vi "Initialize AO Channels.vi"(8 "error in (no error)":errorcluster, 11 "Instrument.Lockin":refnum<class "Instrument.Lockin.lvclass">) -> (0 "error out":errorcluster, 3 "Instrument.Lockin out":refnum<class "Instrument.Lockin.lvclass">)   [LabVIEW 2020, in "Instrument.Lockin.lvclass"]
uses:
  Instrument.Lockin.lvclass
  Instrument.Lockin.lvclass/Instrument.Lockin.ctl
  LockinDAQ/Typedefs/Function-enum.ctl
  LockinDAQ/LockinDAQ.lvclass
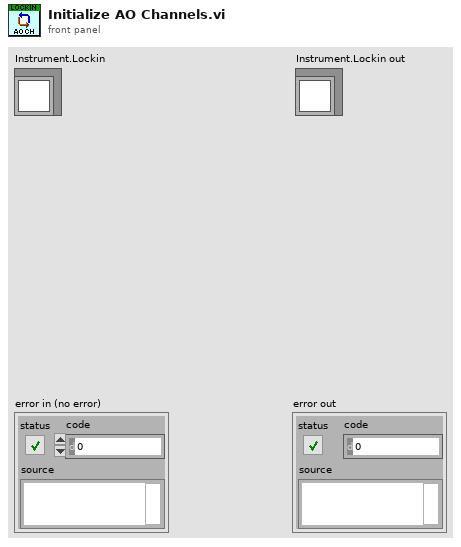
[diagram p1: front panel]
types:
  T1 = typedef "LockinDAQ.lvclass/AO-cluster.ctl" = cluster{"Ch":i32[], "Amp (V)":dbl[], "DC (V)":dbl[], "f (Hz)":dbl[], "Phase (°)":dbl[], "Function":T2[], "Sweep?":bool[]}
  T2 = typedef "LockinDAQ.lvclass/Function-enum.ctl" = enum16{"Sine", "Triangle", "Square", "Sawtooth"}
  T3 = typedef "LockinDAQ.lvclass/AO.config-array.ctl" = T4[]
  T4 = typedef "LockinDAQ.lvclass/AO.config-cluster.ctl" = cluster{"AO.channels":tag, "AO.Range":T5, "output terminal configuration":i32, "DAQ Type":T6}
  T5 = typedef "LockinDAQ.lvclass/446xAO-enum.ctl" = enum16{"±0.1 V", "±1.0 V", "±10.0 V"}
  T6 = typedef "LockinDAQ.lvclass/DAQType-enum.ctl" = enum16{"None", "USB 4431", "PXI 446x"}
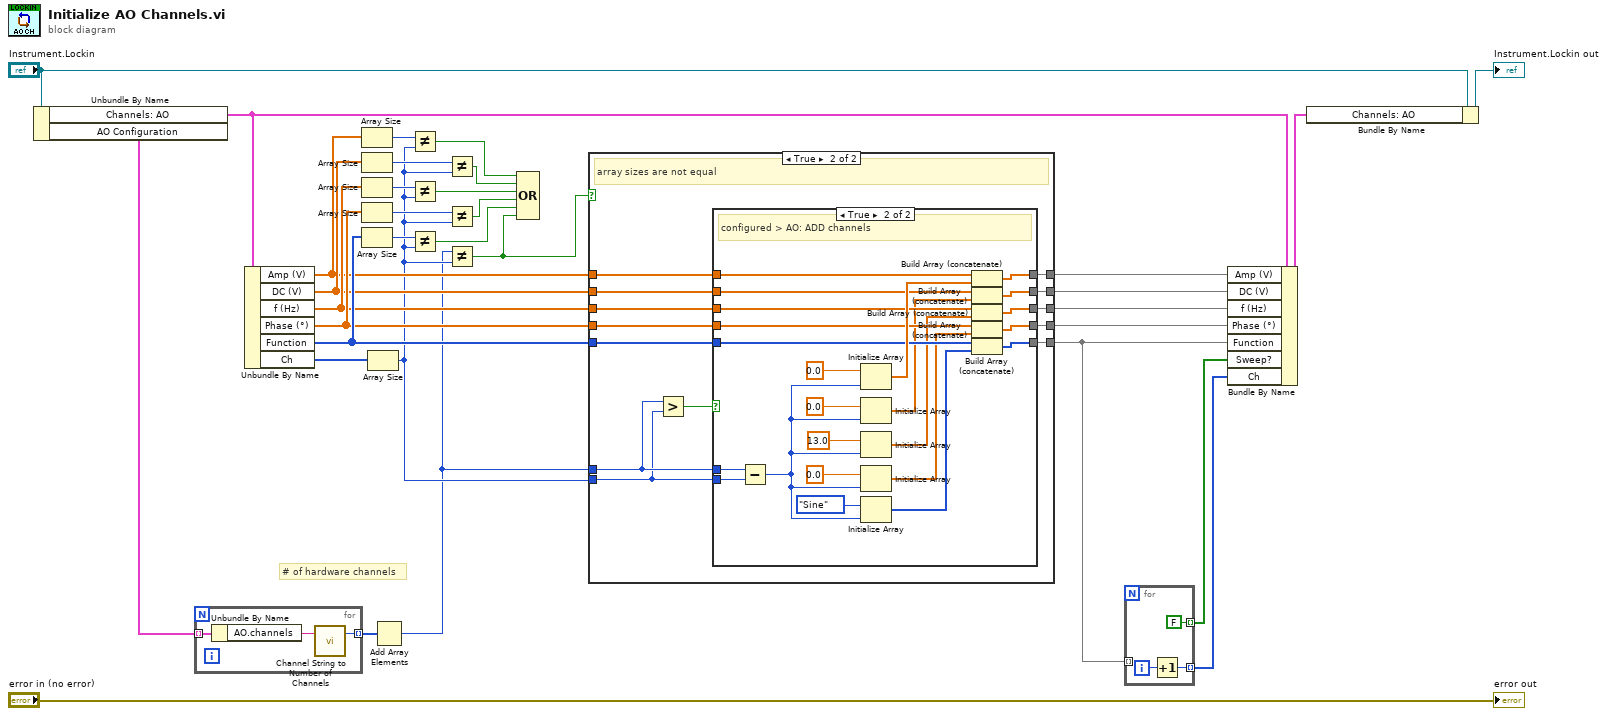
[diagram p0: block diagram]
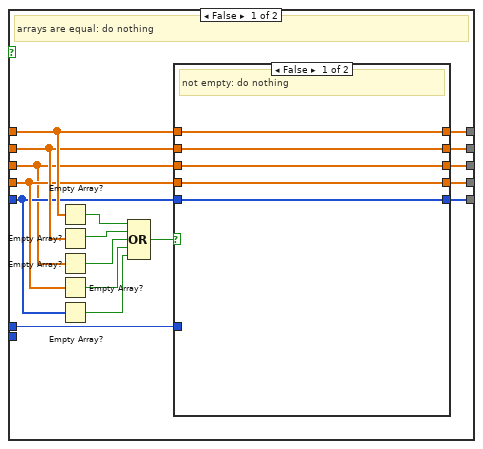
[diagram p2: hidden frame]
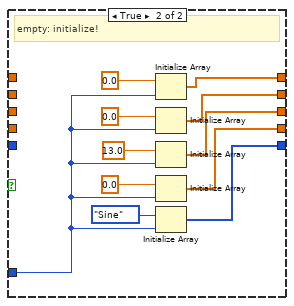
[diagram p3: hidden frame]
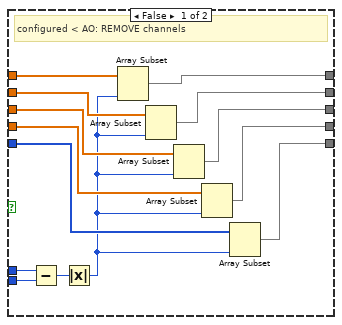
[diagram p4: hidden frame]
diagram:
  # "# of hardware channels"
  n1 = Unbundle By Name("Instrument.Lockin") -> ("Channels: AO"=w28:T1, "AO Configuration"=w5:T3)
  n2 = for {
    tunnel: w5 -> [w36] mode=indexing
    tunnel: [w35] -> w30 mode=indexing
    n3 = Unbundle By Name(w36) -> ("AO.channels"=w34:tag)
    n4 = call "Channel String to Number of Channels.vi"("Channels String"=w34) -> ("# channels"=w35:i32)  [unwired: 2 in]
  }
  n5 = Unbundle By Name(w28) -> ("Amp (V)"=w20:dbl[], "DC (V)"=w21:dbl[], "f (Hz)"=w22:dbl[], "Phase (°)"=w23:dbl[], "Function"=w24:T2[], "Ch"=w8:i32[])
  n6 = Array Size(array=w20) -> (size(s)=w19:i32)
  n7 = Array Size(array=w21) -> (size(s)=w18:i32)
  n8 = Array Size(array=w22) -> (size(s)=w17:i32)
  n9 = Array Size(array=w23) -> (size(s)=w16:i32)
  n10 = Array Size(array=w24) -> (size(s)=w15:i32)
  n11 = Array Size(array=w8) -> (size(s)=w9:i32)
  n12 = Add Array Elements(numeric array=w30) -> (sum=w4:i32)
  n13 = Not Equal?(x=w19, y=w9) -> (x != y?=w14:bool)
  n14 = Not Equal?(x=w17, y=w9) -> (x != y?=w12:bool)
  n15 = Not Equal?(x=w15, y=w9) -> (x != y?=w10:bool)
  n16 = Not Equal?(x=w18, y=w9) -> (x != y?=w13:bool)
  n17 = Not Equal?(x=w16, y=w9) -> (x != y?=w11:bool)
  n18 = Not Equal?(x=w4, y=w9) -> (x != y?=w3:bool)
  n19 = Compound Arithmetic op=OR(w14, w13, w12, w11, w10, w3) -> ()  [unwired: 1 out]
  n20 = case shown="True" w3 {
    tunnel: [w48 w75] -> w2
    tunnel: w24 -> [w42 w70]
    tunnel: [w49 w76] -> w31
    tunnel: [w47 w74] -> w32
    tunnel: w22 -> [w41 w78]
    tunnel: w21 -> [w44 w80]
    tunnel: [w45 w82] -> w33
    tunnel: w23 -> [w43 w77]
    tunnel: w20 -> [w53 w81]
    tunnel: w4 -> [w50 w72]
    tunnel: w9 -> [_ w71]
    tunnel: [w46 w79] -> w27
    frame False {
      # "arrays are equal: do nothing"
      n21 = Empty Array?(array=w53) -> (empty?=w52:bool)
      n22 = Empty Array?(array=w44) -> (empty?=w40:bool)
      n23 = Empty Array?(array=w41) -> (empty?=w39:bool)
      n24 = Empty Array?(array=w43) -> (empty?=w38:bool)
      n25 = Empty Array?(array=w42) -> (empty?=w37:bool)
      n26 = Compound Arithmetic op=OR(w52, w40, w39, w38, w37) -> (w51:bool)
      n27 = case shown="False" w51 {
        tunnel: w42 -> [w54 _]
        tunnel: w43 -> [w55 _]
        tunnel: w41 -> [w56 _]
        tunnel: w44 -> [w57 _]
        tunnel: w53 -> [w58 _]
        tunnel: w50 -> [_ w64]
        tunnel: [w55 w63] -> w49
        tunnel: [w54 w62] -> w48
        tunnel: [w56 w61] -> w47
        tunnel: [w57 w60] -> w46
        tunnel: [w58 w59] -> w45
        frame False {
          # "not empty: do nothing"
        }
        frame True {
          # "empty: initialize!"
          n28 = Initialize Array(0.0, w64) -> (w59:dbl[])
          n29 = Initialize Array(0.0, w64) -> (w60:dbl[])
          n30 = Initialize Array(13.0, w64) -> (w61:dbl[])
          n31 = Initialize Array(0.0, w64) -> (w63:dbl[])
          n32 = Initialize Array(Function-enum."Sine" ("Signal Type"), w64) -> (w62:T2[])
        }
      }
    }
    frame True {
      # "array sizes are not equal"
      n33 = Greater?(x=w72, y=w71) -> (0:w73:bool)
      n34 = case shown="True" w73 {
        tunnel: [w91 w114] -> w82
        tunnel: w81 -> [w92 w113]
        tunnel: w72 -> [w86 w111]
        tunnel: w71 -> [w85 w110]
        tunnel: w80 -> [w93 w108]
        tunnel: [w90 w107] -> w79
        tunnel: w78 -> [w94 w106]
        tunnel: w77 -> [w95 w105]
        tunnel: [w88 w104] -> w76
        tunnel: [w87 w102] -> w75
        tunnel: [w89 w97] -> w74
        tunnel: w70 -> [w96 w103]
        frame False {
          # "configured < AO: REMOVE channels"
          n35 = Subtract(x=w86, y=w85) -> (x-y=w84:i32)
          n36 = Absolute Value(x=w84) -> (abs(x)=w83:i32)
          n37 = Array Subset(array=w92, length=w83) -> (w91:dbl[])  [unwired: 1 in]
          n38 = Array Subset(array=w93, length=w83) -> (w90:dbl[])  [unwired: 1 in]
          n39 = Array Subset(array=w94, length=w83) -> (w89:dbl[])  [unwired: 1 in]
          n40 = Array Subset(array=w95, length=w83) -> (w88:dbl[])  [unwired: 1 in]
          n41 = Array Subset(array=w96, length=w83) -> (w87:T2[])  [unwired: 1 in]
        }
        frame True {
          # "configured > AO: ADD channels"
          n42 = Subtract(x=w111, y=w110) -> (x-y=w109:i32)
          n43 = Initialize Array(0.0, w109) -> (w112:dbl[])
          n44 = Initialize Array(0.0, w109) -> (w101:dbl[])
          n45 = Initialize Array(13.0, w109) -> (w100:dbl[])
          n46 = Initialize Array(0.0, w109) -> (w99:dbl[])
          n47 = Initialize Array(Function-enum."Sine" ("Signal Type"), w109) -> (w98:T2[])
          n48 = Build Array (concatenate)(w113, w112) -> (w114:dbl[])
          n49 = Build Array (concatenate)(w108, w101) -> (w107:dbl[])
          n50 = Build Array (concatenate)(w106, w100) -> (w97:dbl[])
          n51 = Build Array (concatenate)(w105, w99) -> (w104:dbl[])
          n52 = Build Array (concatenate)(w103, w98) -> (w102:T2[])
        }
      }
    }
  }
  n53 = for {
    tunnel: [w121] -> w7 mode=indexing
    tunnel: w2 -> [_] mode=indexing
    tunnel: [FALSE] -> w1 mode=indexing
    i -> [w122]
    n54 = Increment(x=w122) -> (x+1=w121:i32)
  }
  n55 = Bundle By Name(cluster=w28, "Amp (V)"=w33, "DC (V)"=w27, "f (Hz)"=w32, "Phase (°)"=w31, "Function"=w2, "Sweep?"=w1, "Ch"=w7) -> (w6:T1)
  n56 = Bundle By Name(cluster="Instrument.Lockin", "Channels: AO"=w6) -> (→"Instrument.Lockin out":refnum<class "Instrument.Lockin.lvclass">)
  "error out" <- "error in (no error)"
